vi "Error log.vi"(8 "error in (no error)":errorcluster) -> (0 "error in (no error) 2":errorcluster)   [LabVIEW 2018]
uses:
  Error log/Error log.lvclass
  C:/Users/observer/Desktop/SPARC4_ACS/SPARC4_ACS/Log File/Log File.lvclass
  Log File/Log File.lvclass/Log File.ctl
  <vilib>/addons/_JKI Toolkits/Caraya/classes/Assert/Assert Equal Value_Variant.vi
  <vilib>/addons/_JKI Toolkits/Caraya/classes/Assert/Assert Not Error.vi
  <vilib>/addons/_JKI Toolkits/Caraya/classes/Test/Test.lvclass
  Log File/Log File.lvclass
  <vilib>/addons/_JKI Toolkits/Caraya/classes/Assert/Assert.lvclass
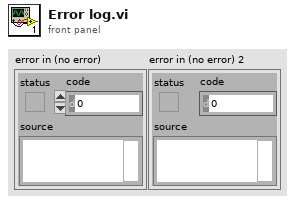
[diagram p1: front panel]
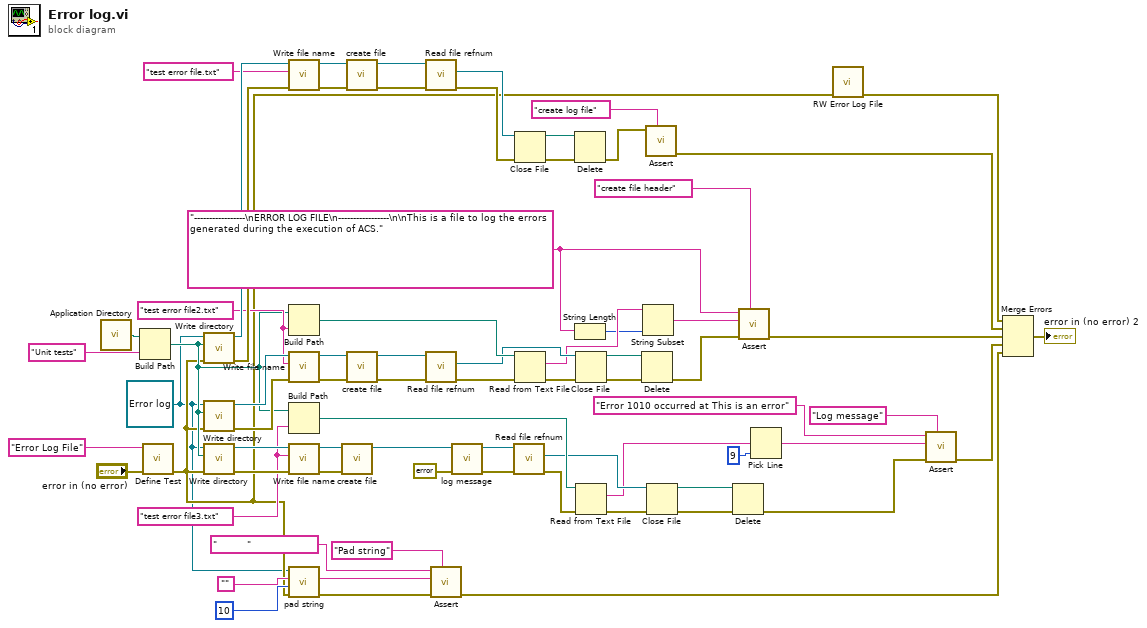
[diagram p0: block diagram]
diagram:
  w1 = "-----------------\nERROR LOG FILE\n-----------------\n\nThis is a file to log the errors generated during the execution of ACS." ("message of the file header")
  w7 = refnum<class "Error log.lvclass"> refnum ("Error log.lvclass")
  w30 = "test error file3.txt" ("file name")
  w45 = "test error file2.txt" ("file name")
  n1 = call <vilib>:"Application Directory.vi"() -> ("Application Directory"=w66:path)
  n2 = Build Path(base path=w66, name or relative path="Unit tests") -> (appended path=w29:path)
  n3 = call <vilib>:"Define Test.vi"("error in (no error)"="error in (no error)", "Label (VI Title)"="Error Log File") -> ("error out"=w8:errorcluster)  [unwired: 8 in, 1 out]
  n4 = call "Write directory.vi"("error in (no error)"=w8, "directory"=w29, "Log File in"=w7) -> ("error out"=w68:errorcluster, "Log File out"=w67:refnum<class "Error log.lvclass">)  [unwired: 7 in]
  n5 = call "Write directory.vi"("error in (no error)"=w8, "directory"=w29, "Log File in"=w7) -> ("error out"=w52:errorcluster, "Log File out"=w51:refnum<class "Error log.lvclass">)  [unwired: 7 in]
  n6 = call "Write directory.vi"("error in (no error)"=w8, "directory"=w29, "Log File in"=w7) -> ("error out"=w35:errorcluster, "Log File out"=w34:refnum<class "Error log.lvclass">)  [unwired: 7 in]
  n7 = call "Write file name.vi"("error in (no error)"=w68, "file name"="test error file.txt", "Log File in"=w67) -> ("error out"=w53:errorcluster, "Log File out"=w54:refnum<class "Error log.lvclass">)  [unwired: 7 in]
  n8 = Build Path(base path=w29, name or relative path=w45) -> (appended path=w44:path)
  n9 = call "Write file name.vi"("error in (no error)"=w52, "file name"=w45, "Log File in"=w51) -> ("error out"=w49:errorcluster, "Log File out"=w50:refnum<class "Error log.lvclass">)  [unwired: 7 in]
  n10 = Build Path(base path=w29, name or relative path=w30) -> (appended path=w31:path)
  n11 = call "Write file name.vi"("error in (no error)"=w35, "file name"=w30, "Log File in"=w34) -> ("error out"=w36:errorcluster, "Log File out"=w33:refnum<class "Error log.lvclass">)  [unwired: 7 in]
  n12 = call "pad string.vi"("error in (no error)"=w8, "string size"=u16 10, "input string"="", "Log File in"=w7) -> ("error out"=w9:errorcluster, "output string"=w13:string)  [unwired: 5 in, 1 out]
  n13 = call "create file.vi"("error in (no error)"=w36, "Log File in"=w33) -> ("Log File out"=w32:refnum<class "Error log.lvclass">)  [unwired: 8 in, 1 out]
  n14 = call "create file.vi"("error in (no error)"=w53, "Log File in"=w54) -> ("error out"=w56:errorcluster, "Log File out"=w55:refnum<class "Error log.lvclass">)  [unwired: 8 in]
  n15 = call "create file.vi"("error in (no error)"=w49, "Log File in"=w50) -> ("error out"=w48:errorcluster, "Log File out"=w47:refnum<class "Error log.lvclass">)  [unwired: 8 in]
  n16 = call "Read file refnum.vi"("error in (no error)"=w56, "Log File in"=w55) -> ("error out"=w60:errorcluster, "file refnum"=w57:refnum<file>)  [unwired: 7 in, 1 out]
  n17 = call "Read file refnum.vi"("error in (no error)"=w48, "Log File in"=w47) -> ("error out"=w46:errorcluster, "file refnum"=w37:refnum<file>)  [unwired: 7 in, 1 out]
  n18 = call-poly <vilib>:"Assert.vi"("Label"="Pad string" ("Label (VI Title)"), "error in (no error)"=w9, "Y"=w13, "X"="          ") -> ("error out"=w10:errorcluster)  [unwired: 6 in, 1 out]
  n19 = call-dynamic "log message.vi"("error in (no error)"=errorcluster {"status"=TRUE, "code"=1010, "source"="This is an error"} ("error in (no error) 3"), "Error log in"=w32) -> ("error out"=w22:errorcluster, "Error log out"=w21:refnum<class "Error log.lvclass">)  [unwired: 8 in]
  n20 = call "Read file refnum.vi"("error in (no error)"=w22, "Log File in"=w21) -> ("error out"=w20:errorcluster, "file refnum"=w19:refnum<file>)  [unwired: 7 in, 1 out]
  n21 = Close File(refnum=w57, error in=w60) -> (path=w58:path, error out=w59:errorcluster)
  n22 = Read from Text File(file (use dialog)=w44, error in=w46) -> (text=w3:string, error out=w41:errorcluster)  [unwired: 2 in, 2 out]
  n23 = Delete(path (use dialog)=w58, error in=w59) -> (error out=w64:errorcluster)  [unwired: 3 in, 2 out]
  n24 = String Length(string=w1) -> (length=w2:i32)
  n25 = Close File(refnum=w37, error in=w41) -> (path=w39:path, error out=w42:errorcluster)
  n26 = Read from Text File(file (use dialog)=w31, error in=w20) -> (text=w17:string, error out=w26:errorcluster)  [unwired: 2 in, 2 out]
  n27 = Delete(path (use dialog)=w39, error in=w42) -> (error out=w40:errorcluster)  [unwired: 3 in, 2 out]
  n28 = String Subset(string=w3, length (rest)=w2) -> (substring=w4:string)  [unwired: 1 in]
  n29 = call-poly <vilib>:"Assert.vi"("Label"="create log file" ("Label (VI Title)"), "Not Error?"=w64) -> ("error out"=w63:errorcluster)  [unwired: 8 in, 1 out]
  n30 = Close File(refnum=w19, error in=w26) -> (path=w28:path, error out=w27:errorcluster)
  n31 = Delete(path (use dialog)=w28, error in=w27) -> (error out=w24:errorcluster)  [unwired: 3 in, 2 out]
  n32 = call-poly <vilib>:"Assert.vi"("Label"="create file header" ("Label (VI Title)"), "error in (no error)"=w40, "Y"=w4, "X"=w1) -> ("error out"=w43:errorcluster)  [unwired: 6 in, 1 out]
  n33 = Pick Line(multi-line string=w17, line index=9) -> (output string=w5:string)  [unwired: 1 in]
  n34 = call "RW Error Log File.vi"("error in (no error)"=w8) -> ("error in (no error) 2"=w69:errorcluster)  [unwired: 10 in]
  n35 = call-poly <vilib>:"Assert.vi"("Label"="Log message" ("Label (VI Title)"), "error in (no error)"=w24, "Y"=w5, "X"="Error 1010 occurred at This is an error" ("Label (VI Title)")) -> ("error out"=w25:errorcluster)  [unwired: 6 in, 1 out]
  n36 = Merge Errors(w69, w63, w43, w25, w10) -> (→"error in (no error) 2":errorcluster)
